vi "Continuous Serial Write and Read.vi"() -> ()   [LabVIEW 2020]
doc: "This example performs writes and reads on a serial port, as directed by the user. You can press the Write and Read buttons, and change the Read Count, while the example is running.\n\nThe parameters set for the serial port must match the parameters of the connected instrument or device. In this example, the Read Count parameter specifies the number of bytes that the serial port reads. If there were more bytes at the port than the specified number, those bytes would not be read. If there were less bytes at the port than the specified number, you would receive a timeout error.\n\nThis example expands upon the flow control options for XON and XOFF, allowing the user to choose those control characters. Also, the user can enable or disable a termination character. Some devices require a termination character in order to identify the end of command strings. Some devices send a termination character to signify the end of data to be read. This example shows how you can end the Read operation once a termination character is detected in the buffer and/or append a termination character at the end of the Write data."
uses:
  Program Files/National Instruments/LabVIEW 2020/examples/Instrument IO/Serial/support/Serial - Settings.ctl
  <vilib>/Instr/_visa.llb/VISA Configure Serial Port (Instr).vi
panel:
  in  "Stop 2":bool
  in  "Termination Character":u8=13 format="%.0x"
  in  "End Write on Termination Character?":bool=TRUE
  in  "Command":string="L6O1"
  in  "Read Count":u32=1000
  out "Response":string="l6F131.122P22.5S1\n\rl6F131.122P18.4S1\n\rl6F131.122P-4.5S1\n\rl6F131.122P-0.4S1\n\rl6F131.122P-0.4S1\n\rl6F131.122P8.7S1\n\rl6F131.122P13.1S1\n\rl6F131.122P22.5S1\n\rl6F131.122P22.5S0\n\rl6F131.122P22.5S0\n\rl6F131.122P22.5S0\n\rl6F131.122P22.5S0\n\rl6F131.122P22.5S0\n\rl6F131.122P22.5S1\n\rl6F131.122P22.5S0\n\rl6F131.122P-8.8S0\n\rl6F131.122P-8.8S0\n\rl6F131.122P22.5S0\n\rl6F131.122P16.9S1\n\rl6F131.122P22.5S1\n\rl6F131.122P22.5S0\n\rl6F131.122P22.5S1\n\rl6F131.122P22.5S1\n\rl6F131.122P22.5S1\n\rl6F131.122P22.5S1\n\rl6F131.122P22.5S1\n\rl6F131.122P22.5S1\n\rl6F131.122P22.5S1\n\rl6F131.122P-8.5S1\n\rl6F131.122P-8.5S0\n\r"
  in  "Write":bool
  in  "Serial Settings":T1={"baud rate"=57600, "data bits"=8, "parity"=enum."None", "stop bits"=10, "flow control"=0} {"flow control" items=["None"=0, "XON/XOFF"=1, "RTS/CTS"=2, "DTR/DSR"=4]; "stop bits" items=["1.0"=10, "1.5"=15, "2.0"=20]; "data bits" min=5 max=8 step=1; "baud rate" items=["75"=75, "110"=110, "134"=134, "150"=150, "300"=300, "600"=600, "1200"=1200, "1800"=1800, "2400"=2400, "4800"=4800, "7200"=7200, "9600"=9600, "14400"=14400, "19200"=19200, "28800"=28800, "38400"=38400, "56000"=56000, "57600"=57600, "115200"=115200, "128000"=128000, "230400"=230400]}
  in  "End Read on Termination Character?":bool=TRUE
  in  "VISA resource name":refnum<visa-resource-name>="COM3"
  # "Overview: Demonstrates the use of the VISA functions to write commands to and read responses from a serial instrument continuously in a loop.\nRequirements: NI-VISA Driver\nInstructions:\n1. Run the VI.\n2. Specify a Command and click the Write button.\n3. Read a Response by clicking the Read button.\n4. Click Stop to stop the VI."
  # "0xA is equivalent to a '\\n' character, which is a line feed."
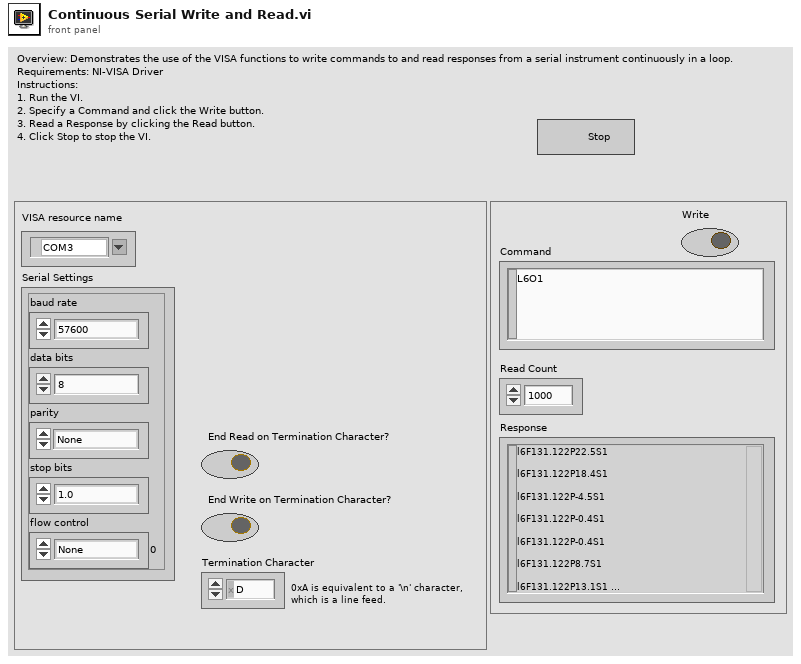
[diagram p1: front panel]
types:
  T1 = typedef "Serial - Settings.ctl" = cluster{"baud rate":u32, "data bits":u16, "parity":enum16{"None", "Odd", "Even", "Mark", "Space"}, "stop bits":u16, "flow control":u16}
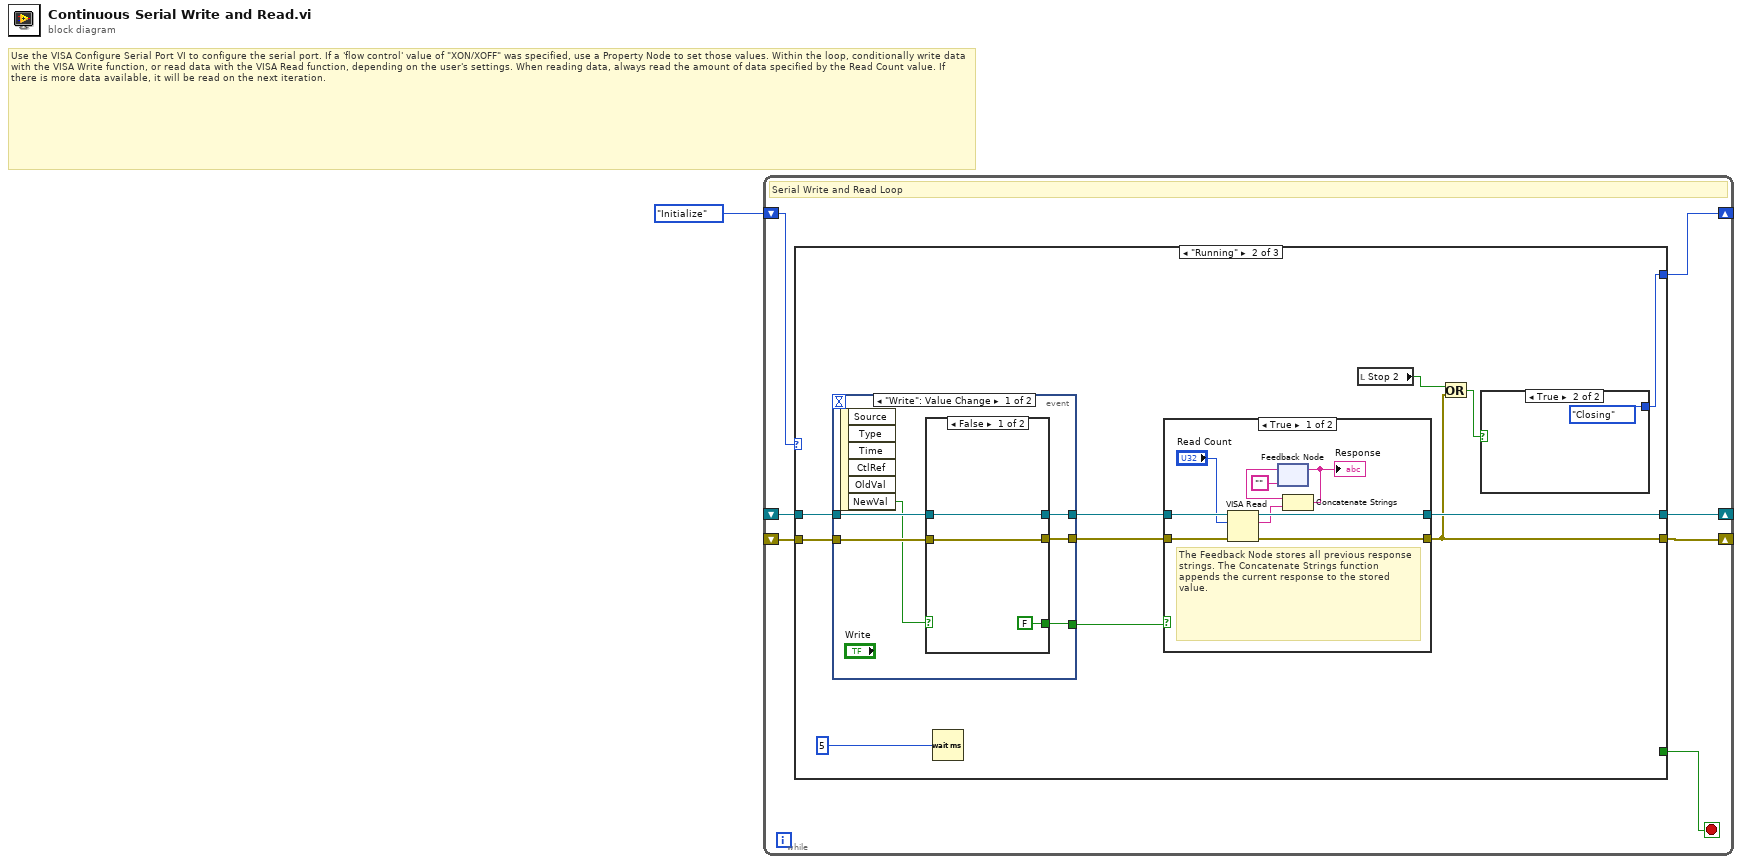
[diagram p0: block diagram]
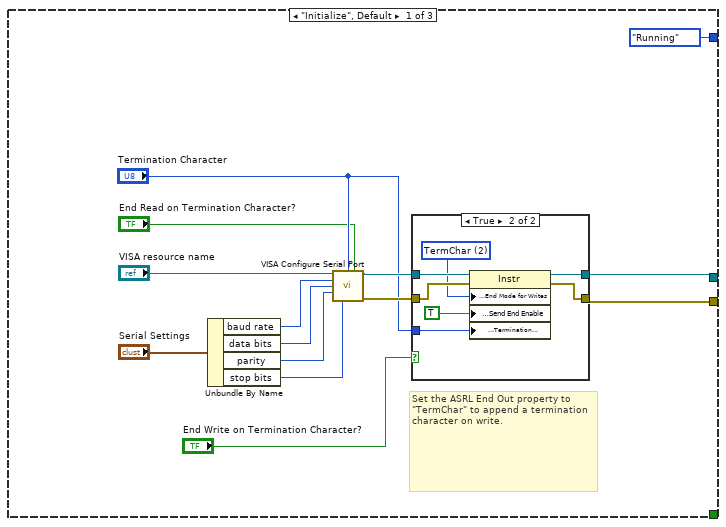
[diagram p2: hidden frame]
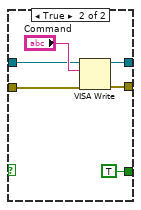
[diagram p4: hidden frame]
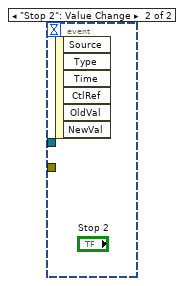
[diagram p5: hidden frame]
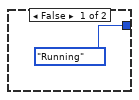
[diagram p6: hidden frame]
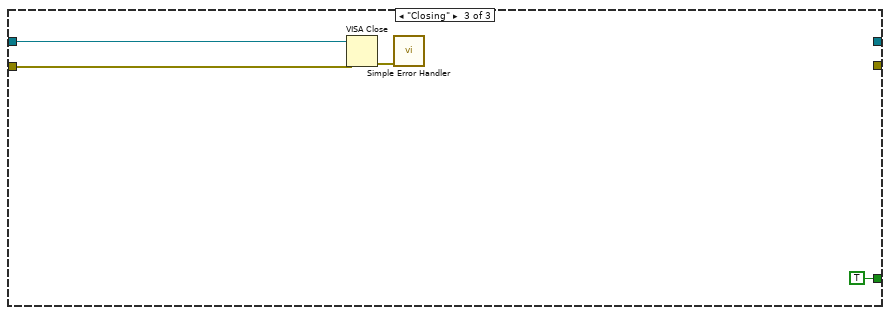
[diagram p8: hidden frame]
diagram:
  # "Use the VISA Configure Serial Port VI to configure the serial port. If a 'flow control' value of \"XON/XOFF\" was specified, use a Property Node to set those values. Within the loop, conditionally write data with the VISA Write function, or read data with the VISA Read function, depending on the user's settings. When reading data, always read the amount of data specified by the Read Count value. If there is more data available, it will be read on the next iteration."
  n1 = while {
    shift-right: [w8] -> _
    shift-left: _ -> [w7]
    shift-right: [w4] -> _
    shift-left: enum16{"Initialize", "Running", "Closing"}."Initialize" -> [w5]
    shift-right: [w6] -> _
    shift-left: _ -> [w3]
    stop <- w2 stop-if-true
    # "Serial Write and Read Loop"
    n2 = case shown="\"Running\"" w5 {
      tunnel: [w11 w42 _] -> w8
      tunnel: w7 -> [_ w41 w73]
      tunnel: [w10 w37 _] -> w6
      tunnel: [enum16{"Initialize", "Running", "Closing"}."Running" w36 _] -> w4
      tunnel: w3 -> [_ w35 w72]
      tunnel: [_ _ TRUE] -> w2
      frame "Initialize", Default {
        # "Set the ASRL End Out property to \"TermChar\" to append a termination character on write."
        n3 = Unbundle By Name("Serial Settings") -> ("baud rate"=w16:u32, "data bits"=w15:u16, "parity"=w14:enum16{"None", "Odd", "Even", "Mark", "Space"}, "stop bits"=w13:u16)
        n4 = call-poly "VISA Configure Serial Port"("VISA resource name"="VISA resource name", "termination char\n(0xA = '\\n' = LF)"="Termination Character", "Enable Termination\nChar (T)"="End Read on Termination Character?", "baud rate (9600)"=w16, "data bits (8)"=w15, "parity (0:none)"=w14, "stop bits (10: 1 bit)"=w13) -> ("VISA resource name out"=w21:refnum<visa-resource-name>, "error out"=w22:errorcluster)  [unwired: 3 in, 4 out]
        n5 = case shown="True" "End Write on Termination Character?" {
          tunnel: w21 -> [w23 w31]
          tunnel: w22 -> [w24 w30]
          tunnel: [w23 w29] -> w11
          tunnel: [w24 w28] -> w10
          tunnel: "Termination Character" -> [_ w26]
          frame False {
          }
          frame True {
            w27 = u16 2 items=["None", "LastBit", "TermChar", "Break"] ("Serial Settings:Serial End Mode for Writes")
            n6 = property class="Instr"(reference=w31, error in=w30, "Serial Settings:End Mode for Writes"=w27, "Message Based Settings:Send End Enable"=TRUE, "Message Based Settings:Termination Character"=w26) -> (reference out=w29:refnum<visa-resource-name>, error out=w28:errorcluster)
          }
        }
      }
      frame "Running" {
        n7 = event shown="[0] \"Write\": Value Change" {
          selector: _ -> [_ _]
          dyn-events: _ -> [_ _]
          timeout: _ -> [_ _]
          tunnel: w41 -> [w48 _]
          tunnel: [w47 _] -> w40
          tunnel: [w46 _] -> w39
          tunnel: w35 -> [w45 _]
          tunnel: [w43 _] -> w32
          event "Write": Value Change {
            n8 = event-data() -> ("NewVal"=w44:bool)  [unwired: 1 in, 5 out]
            n9 = case shown="False" w44 {
              tunnel: w48 -> [w51 w56]
              tunnel: [w51 w55] -> w47
              tunnel: [w50 w54] -> w46
              tunnel: w45 -> [w50 w53]
              tunnel: [FALSE TRUE] -> w43
              frame False {
              }
              frame True {
                n10 = VISA Write(VISA resource name=w56, write buffer="Command", error in (no error)=w53) -> (VISA resource name out=w55:refnum<visa-resource-name>, error out=w54:errorcluster)  [unwired: 1 out]
              }
            }
          }
          event "Stop 2": Value Change {
            n11 = event-data() -> ()  [unwired: 1 in, 6 out]
          }
        }
        n12 = Wait (ms)(milliseconds to wait=u32 5) -> ()  [unwired: 1 out]
        n13 = case shown="True" w32 {
          tunnel: [w66 w70] -> w42
          tunnel: w40 -> [w68 w70]
          tunnel: [w64 w69] -> w37
          tunnel: w39 -> [w67 w69]
          frame True {
            # "The Feedback Node stores all previous response strings. The Concatenate Strings function appends the current response to the stored value."
            n14 = VISA Read(VISA resource name=w68, byte count="Read Count", error in (no error)=w67) -> (VISA resource name out=w66:refnum<visa-resource-name>, read buffer=w63:string, error out=w64:errorcluster)  [unwired: 1 out]
            n15 = feedback #1("") -> (w62:string)
            n16 = Concatenate Strings(w62, w63) -> (w61:string)
            "Response" <- w61
            n17 = feedback-in #1(w61) -> ()
          }
          frame False {
          }
        }
        n18 = local read "Stop 2"() -> (w33:bool)
        n19 = Or(x=w33, y=w37) -> (x .or. y?=w38:bool)
        n20 = case shown="True" w38 {
          tunnel: [enum16{"Initialize", "Running", "Closing"}."Running" enum16{"Initialize", "Running", "Closing"}."Closing"] -> w36
          frame False {
          }
          frame True {
          }
        }
      }
      frame "Closing" {
        n21 = VISA Close(VISA resource name=w73, error in (no error)=w72) -> (error out=w74:errorcluster)
        n22 = call <vilib>:"Simple Error Handler.vi"("error in (no error)"=w74) -> ()  [unwired: 1 in, 8 out]
      }
    }
  }
